vi "initialize_instruments (SubVI).vi"(0 "VISA Refnum in":refnum<visa-resource-name>="GPIB0::10::INSTR", 1 "Sample rate":dbl=1000.0 format="%0.2f", 3 "trig_wfm":bool, 5 "Electrode outupt channels":tag="Dev4/ao0", 7 "make volt file":bool, 9 "volt file path":path, 11 "Use synth?":bool) -> (4 "instrument config":T1, 6 "Volt vs pos array":cluster{dbl, dbl}[](array[cluster]))   [LabVIEW 2014]
uses:
  <vilib>/DAQmx/create/channels.llb/DAQmx Create Channel (AO-Voltage-Basic).vi
  <vilib>/DAQmx/configure/timing.llb/DAQmx Timing (Sample Clock).vi
  <vilib>/Utility/file.llb/Read From Spreadsheet File (DBL).vi
  <resource>/objmgr/daqmx.rc
panel:
  out "SampClk.Rate":dbl
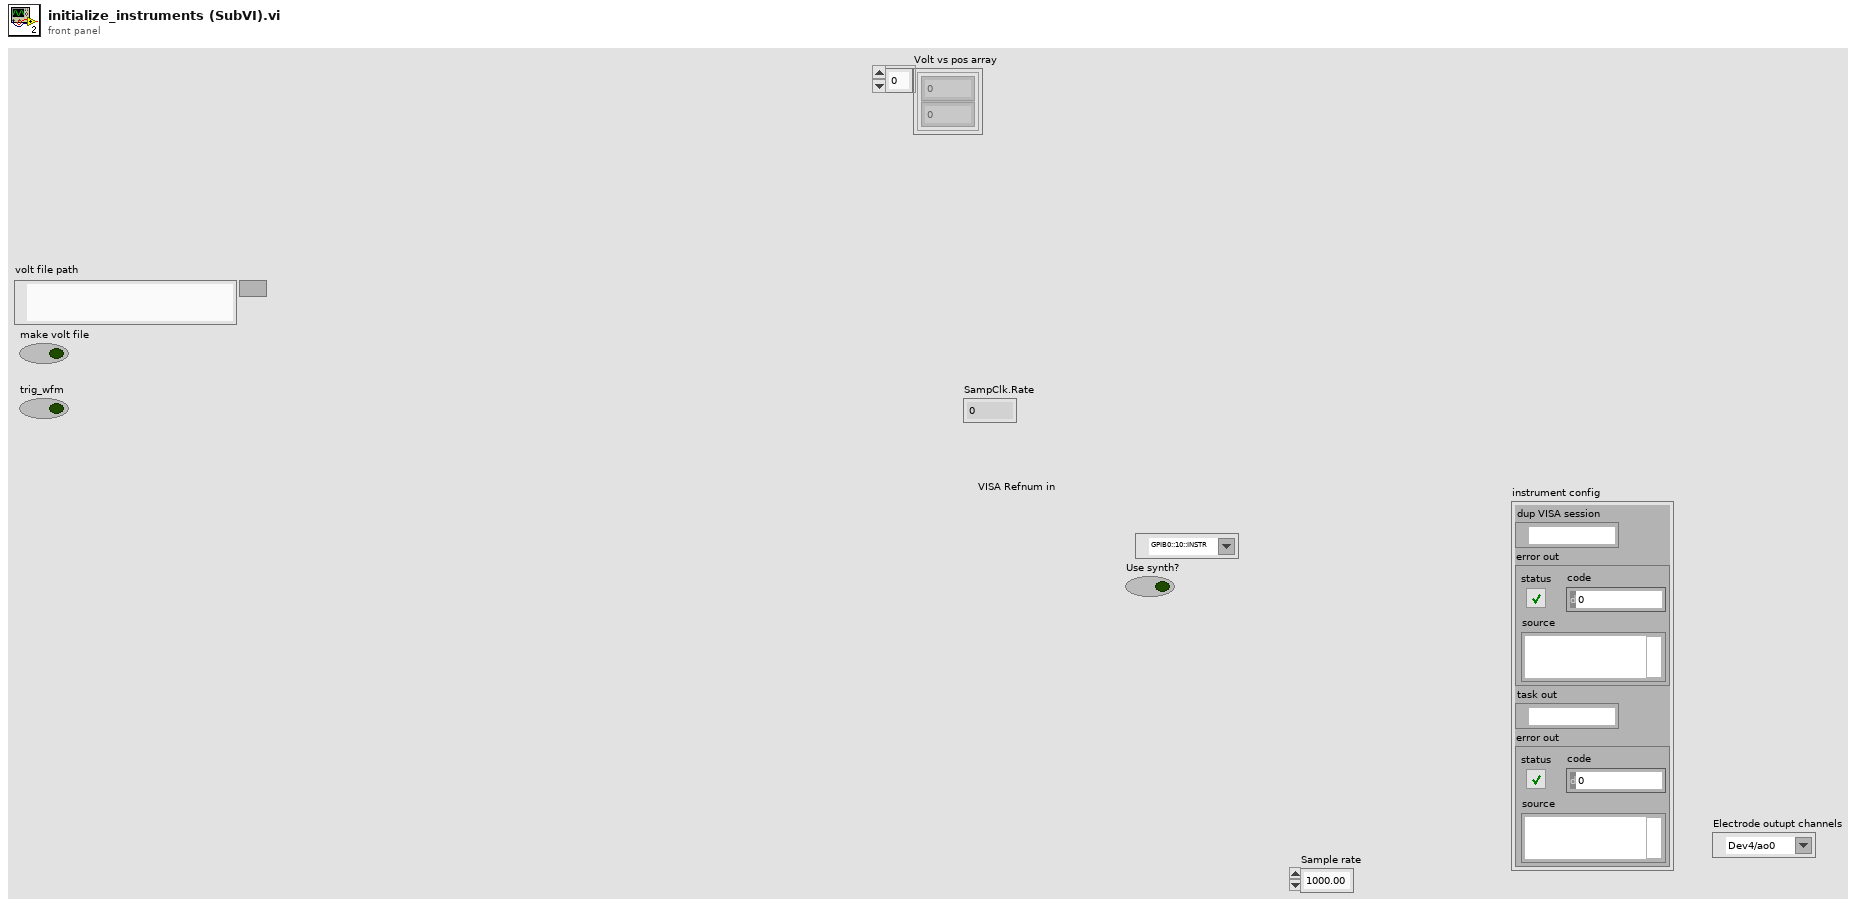
[diagram p1: front panel]
types:
  T1 = cluster{"dup VISA session":refnum<visa-resource-name>, "error out":errorcluster, "task out":refnum<k21>, "error out":errorcluster}
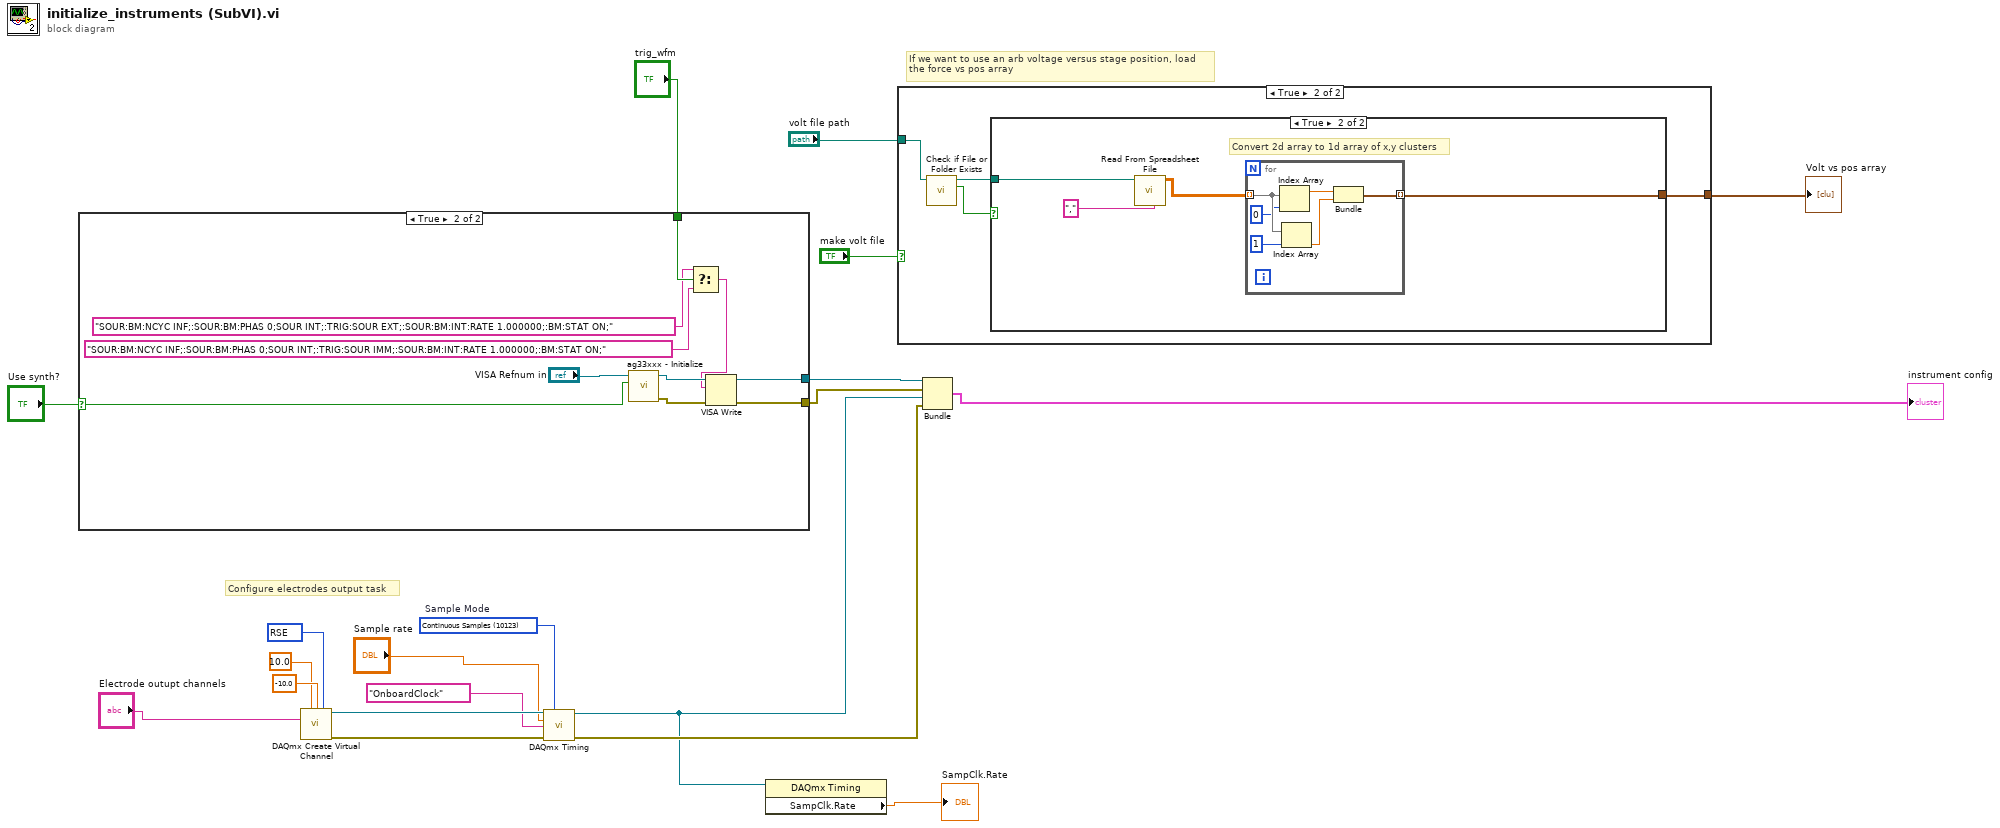
[diagram p0: block diagram]
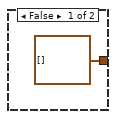
[diagram p2: hidden frame]
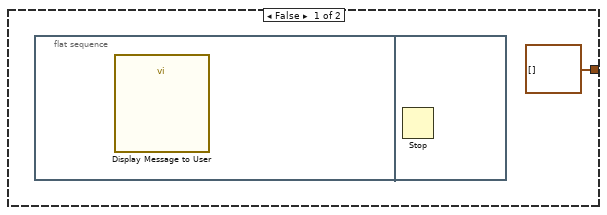
[diagram p3: hidden frame]
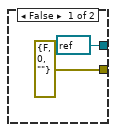
[diagram p4: hidden frame]
diagram:
  w11 = 10083 items=["Default"=-1, "RSE"=10083, "Differential"=10106, "Pseudodifferential"=12529] ("output terminal configuration")
  w17 = 10123 items=["Finite Samples"=10178, "Continuous Samples"=10123, "Hardware Timed Single Point"=12522]  # Sample Mode
  # "If we want to use an arb voltage versus stage position, load\nthe force vs pos array"
  # "Configure electrodes output task"
  n1 = case shown="True" "Use synth?" {
    selector: "Use synth?" -> [_ w27]
    tunnel: [refnum<visa-resource-name> refnum ("dup VISA session") w29] -> w19
    tunnel: [errorcluster {"status"=FALSE, "code"=0, "source"=""} ("error out") w28] -> w18
    tunnel: "trig_wfm" -> [_ w26]
    frame False {
    }
    frame True {
      n2 = call "ag33xxx - Initialize.vi"("ID Query (T: Check)"=w27, "Instrument Resource Name"="VISA Refnum in") -> ("error out"=w31:errorcluster, "dup VISA session"=w30:refnum<visa-resource-name>)  [unwired: 8 in]
      n3 = Select(t="SOUR:BM:NCYC INF;:SOUR:BM:PHAS 0;SOUR INT;:TRIG:SOUR EXT;:SOUR:BM:INT:RATE 1.000000;:BM:STAT ON;" ("write buffer"), s=w26, f="SOUR:BM:NCYC INF;:SOUR:BM:PHAS 0;SOUR INT;:TRIG:SOUR IMM;:SOUR:BM:INT:RATE 1.000000;:BM:STAT ON;" ("write buffer")) -> (s? t:f=w23:string)
      n4 = VISA Write(VISA resource name=w30, write buffer=w23, error in (no error)=w31) -> (VISA resource name out=w29:refnum<visa-resource-name>, error out=w28:errorcluster)  [unwired: 1 out]
    }
  }
  n5 = call-poly <vilib>:"DAQmx Create Virtual Channel.vi"("maximum value"=10.0, "minimum value"=-10.0, "output terminal configuration"=w11, "physical channels"="Electrode outupt channels") -> ("task out"=w15:refnum<k21>, "error out"=w16:errorcluster)  [unwired: 10 in]
  n6 = call-poly <vilib>:"DAQmx Timing.vi"("task/channels in"=w15, "sample mode"=w17, "rate"="Sample rate", "source"=tag "OnboardClock" ("Sample Clock Source"), "error in"=w16) -> ("task out"=w7:refnum<k21>, "error out"=w9:errorcluster)  [unwired: 9 in]
  n7 = property class="DAQmx Timing"(reference=w7) -> ("SampClk.Rate"=→"SampClk.Rate":dbl)  [unwired: 1 in, 2 out]
  n8 = case shown="True" "make volt file" {
    tunnel: "volt file path" -> [_ w36]
    tunnel: [cluster{dbl, dbl}[] [] w34] -> w1
    frame False {
    }
    frame True {
      n9 = call <vilib>:"Check if File or Folder Exists.vi"("path"=w36) -> ("file or folder exists?"=w37:bool, "dup path"=w35:path)  [unwired: 8 in, 1 out]
      n10 = case shown="True" w37 {
        tunnel: w35 -> [_ w41]
        tunnel: [cluster{dbl, dbl}[] [] w39] -> w34
        frame False {
          n11 = flat-sequence {
            frame #0 {
              n12 = call "Display Message to User"() -> ()  [unwired: 10 in, 2 out]
            }
            frame #1 {
              n13 = Stop() -> ()  [unwired: 1 in]
            }
          }
        }
        frame True {
          # "Convert 2d array to 1d array of x,y clusters"
          n14 = call-poly <vilib>:"Read From Spreadsheet File.vi"("delimiter (\\t)"="," ("delimiter (\\t)"), "file path (dialog if empty)"=w41) -> ("all rows"=w40:dbl[][])  [unwired: 5 in, 4 out]
          n15 = for {
            tunnel: w40 -> [w48] mode=indexing
            tunnel: [w43] -> w39 mode=indexing
            n16 = Index Array(array=w48, index=0) -> (element=w45:dbl)
            n17 = Index Array(array=w48, index=1) -> (element=w44:dbl)
            n18 = Bundle(w45, w44) -> (w43:cluster{dbl, dbl})  [unwired: 1 in]
          }
        }
      }
    }
  }
  "Volt vs pos array" <- w1
  n19 = Bundle("dup VISA session"=w19, "error out"=w18, "task out"=w7, "error out"=w9) -> (→"instrument config":T1)  [unwired: 1 in]
